vi "RPi_BME280_Raw_Measures_to_Calibrated_Measures_Conversion.vi"(0 "Raw Measures":T1, 5 "Calibration Coefficients":T2) -> (4 "Calibrated Measures":T3)   [LabVIEW 2020]
doc: "Converts Raw Measures to Calibrated Pressure, Temperature and Humidity Measures.\n\nMIT License\nCopyright (c) 2021 Asper"
uses:
  Type_Def/BME280_Calibration_Coefficients.ctl
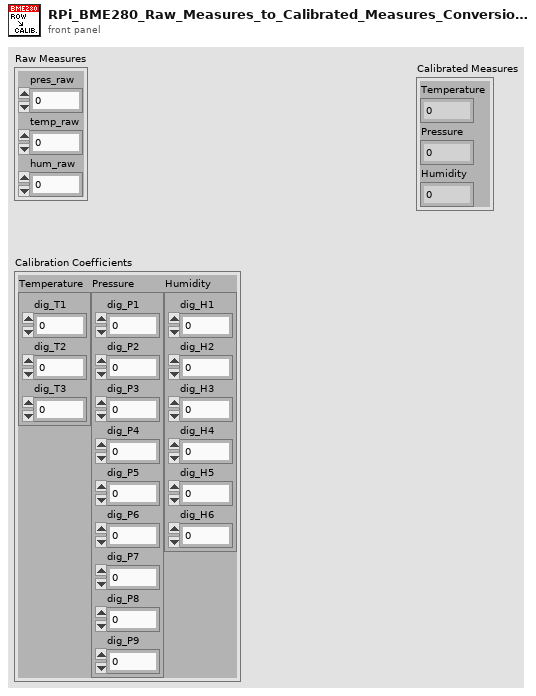
[diagram p1: front panel]
types:
  T1 = cluster{"pres_raw":u32, "temp_raw":u32, "hum_raw":u32}
  T2 = typedef "BME280_Calibration_Coefficients.ctl" = cluster{"Temperature":cluster{"dig_T1":u16, "dig_T2":i16, "dig_T3":i16}, "Pressure":cluster{"dig_P1":u16, "dig_P2":i16, "dig_P3":i16, "dig_P4":i16, "dig_P5":i16, "dig_P6":i16, "dig_P7":i16, "dig_P8":i16, "dig_P9":i16}, "Humidity":cluster{"dig_H1":u8, "dig_H2":i16, "dig_H3":u8, "dig_H4":i16, "dig_H5":i16, "dig_H6":i8}}
  T3 = cluster{"Temperature":dbl, "Pressure":dbl, "Humidity":dbl}
  T4 = cluster{"dig_T1":u16, "dig_T2":i16, "dig_T3":i16}
  T5 = cluster{"dig_H1":u8, "dig_H2":i16, "dig_H3":u8, "dig_H4":i16, "dig_H5":i16, "dig_H6":i8}
  T6 = cluster{"dig_P1":u16, "dig_P2":i16, "dig_P3":i16, "dig_P4":i16, "dig_P5":i16, "dig_P6":i16, "dig_P7":i16, "dig_P8":i16, "dig_P9":i16}
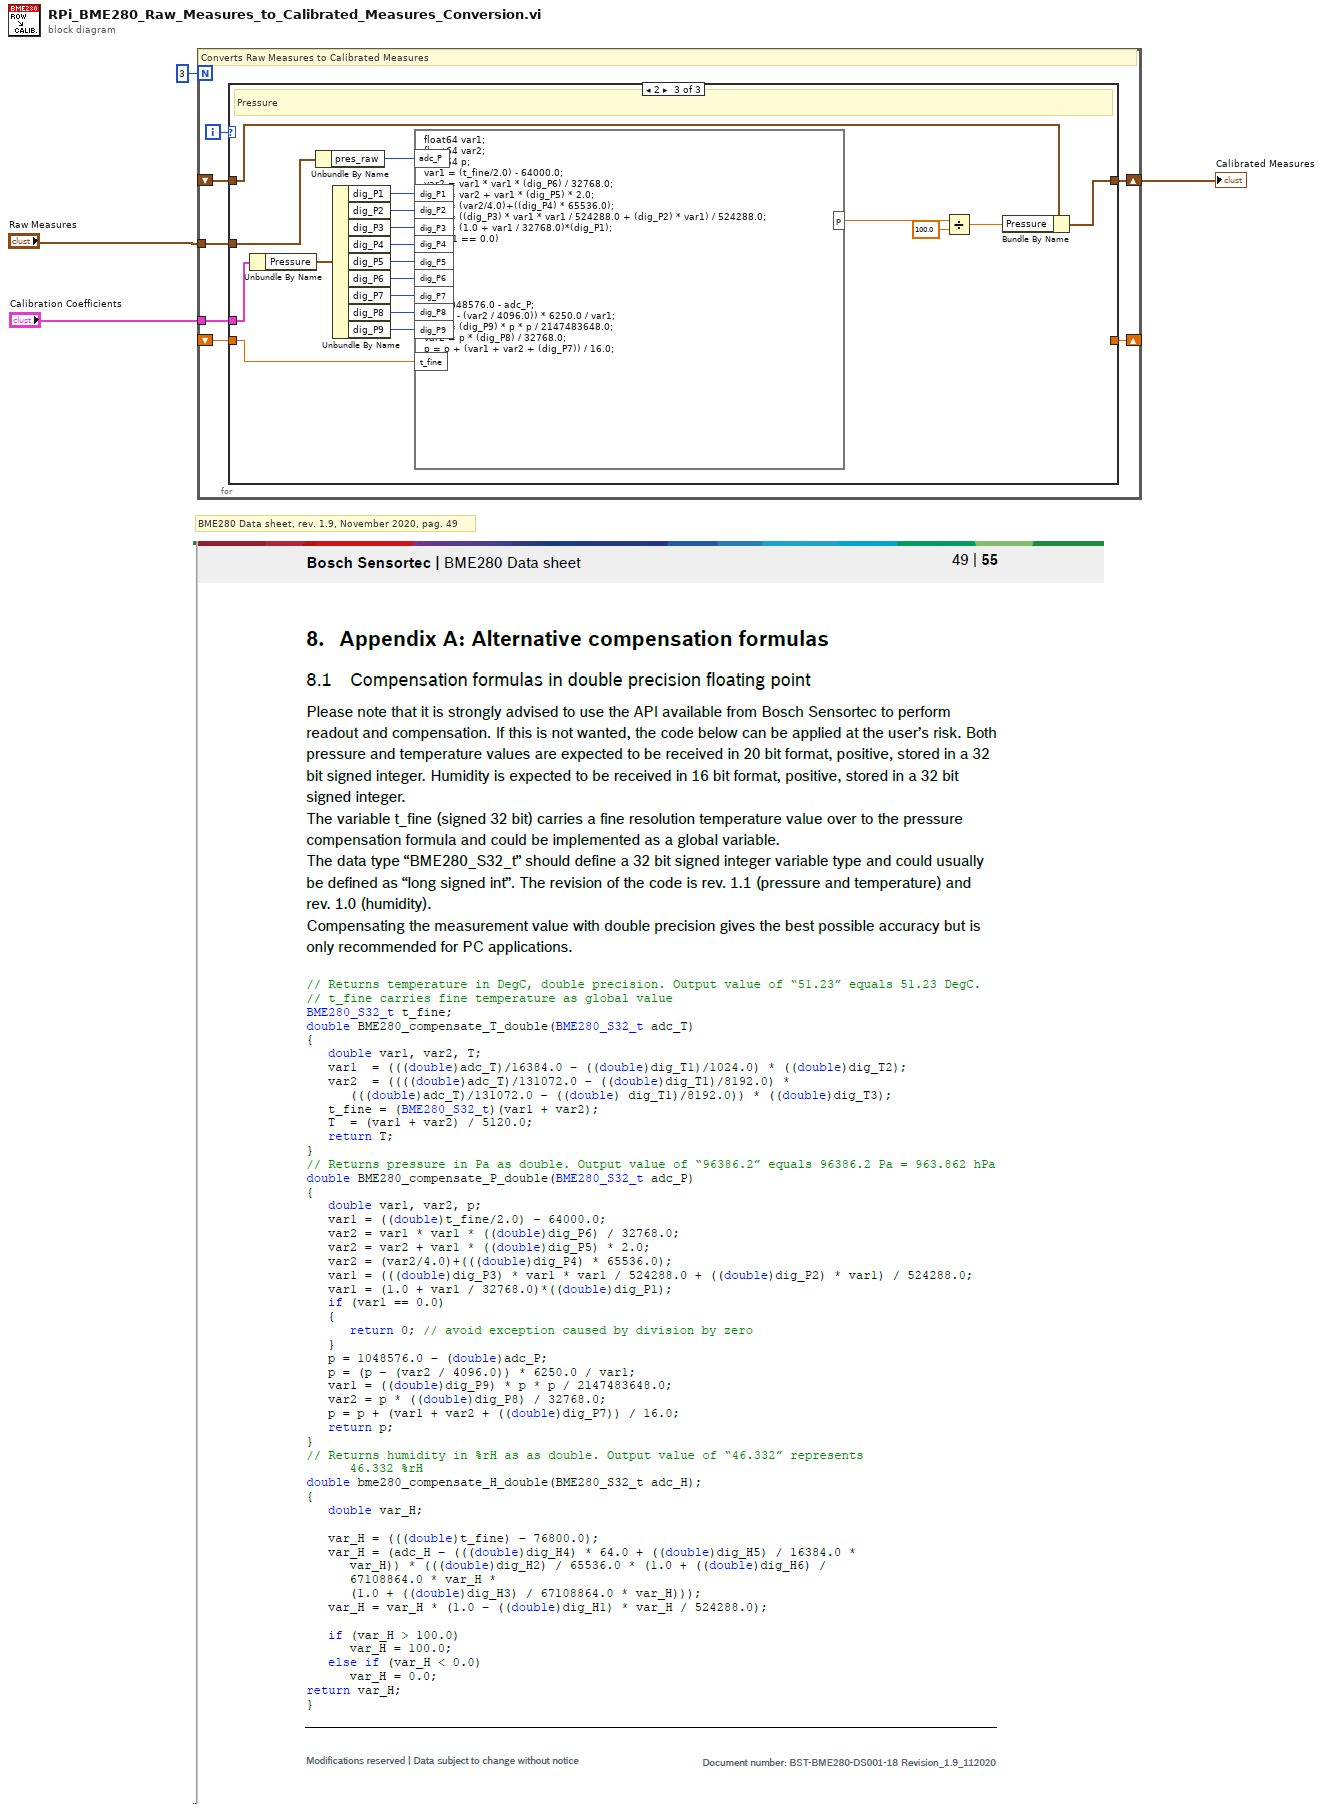
[diagram p0: block diagram]
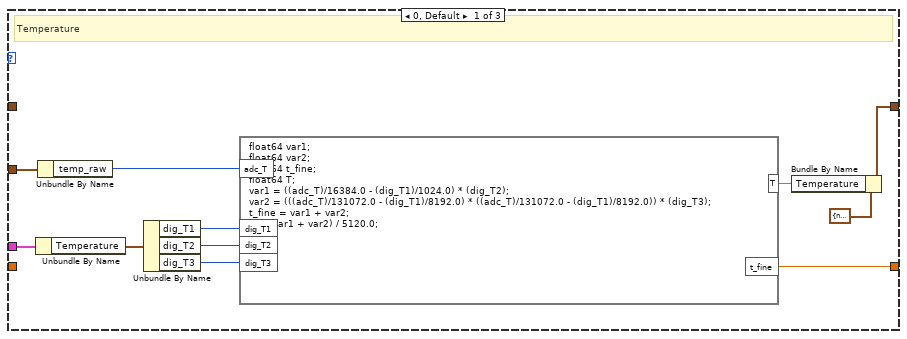
[diagram p2: hidden frame]
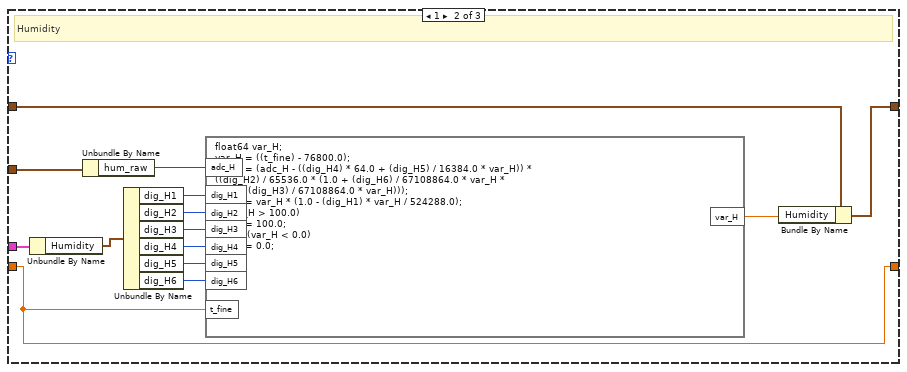
[diagram p3: hidden frame]
diagram:
  # "BME280 Data sheet, rev. 1.9, November 2020, pag. 49"
  n1 = for {
    N: 3 -> [_]
    tunnel: "Raw Measures" -> [w11]
    tunnel: "Calibration Coefficients" -> [w10]
    shift-right: [w8] -> _
    shift-left: _ -> [w7]
    shift-right: [w6] -> w4
    shift-left: _ -> [w5]
    i -> [w9]
    # "Converts Raw Measures to Calibrated Measures"
    n2 = case shown="2" w9 {
      tunnel: w11 -> [w18 w29 w43]
      tunnel: w10 -> [w17 w28 w38]
      tunnel: [w15 w26 _] -> w8
      tunnel: w7 -> [_ w26 w42]
      tunnel: [w12 w23 w39] -> w6
      tunnel: w5 -> [_ w25 w41]
      frame 0, Default {
        # "Temperature"
        n3 = Unbundle By Name(w17) -> ("Temperature"=w16:T4)
        n4 = Unbundle By Name(w18) -> ("temp_raw"=w22:u32)
        n5 = Unbundle By Name(w16) -> ("dig_T1"=w21:u16, "dig_T2"=w20:i16, "dig_T3"=w19:i16)
        n6 = formula code="float64 var1;\nfloat64 var2;\nfloat64 t_fine;\nfloat64 T;\nvar1 = ((adc_T)/16384.0 - (dig_T1)/1024.0) * (dig_T2);\nvar2 = (((adc_T)/131072.0 - (dig_T1)/8192.0) * ((adc_T)/131072.0 - (dig_T1)/8192.0)) * (dig_T3);\nt_fine = var1 + var2;\nT = (var1 + var2) / 5120.0;"("adc_T"=w22, "dig_T1"=w21, "dig_T2"=w20, "dig_T3"=w19) -> ("T"=w13:dbl, "t_fine"=w15:dbl)
        n7 = Bundle By Name(cluster=T3 {"Temperature"=nan, "Pressure"=nan, "Humidity"=nan}, "Temperature"=w13) -> (w12:T3)
      }
      frame 1 {
        # "Humidity"
        n8 = Unbundle By Name(w28) -> ("Humidity"=w27:T5)
        n9 = Unbundle By Name(w29) -> ("hum_raw"=w30:u32)
        n10 = Unbundle By Name(w27) -> ("dig_H1"=w31:u8, "dig_H2"=w32:i16, "dig_H3"=w33:u8, "dig_H4"=w34:i16, "dig_H5"=w35:i16, "dig_H6"=w36:i8)
        n11 = formula code="float64 var_H;\nvar_H = ((t_fine) - 76800.0);\nvar_H = (adc_H - ((dig_H4) * 64.0 + (dig_H5) / 16384.0 * var_H)) *\n((dig_H2) / 65536.0 * (1.0 + (dig_H6) / 67108864.0 * var_H *\n(1.0 + (dig_H3) / 67108864.0 * var_H)));\nvar_H = var_H * (1.0 - (dig_H1) * var_H / 524288.0);\nif (var_H > 100.0)\nvar_H = 100.0;\nelse if (var_H < 0.0)\nvar_H = 0.0;"("adc_H"=w30, "dig_H1"=w31, "dig_H2"=w32, "dig_H3"=w33, "dig_H4"=w34, "dig_H5"=w35, "dig_H6"=w36, "t_fine"=w26) -> ("var_H"=w24:dbl)
        n12 = Bundle By Name(cluster=w25, "Humidity"=w24) -> (w23:T3)
      }
      frame 2 {
        # "Pressure"
        n13 = Unbundle By Name(w38) -> ("Pressure"=w37:T6)
        n14 = Unbundle By Name(w43) -> ("pres_raw"=w45:u32)
        n15 = Unbundle By Name(w37) -> ("dig_P1"=w46:u16, "dig_P2"=w47:i16, "dig_P3"=w48:i16, "dig_P4"=w49:i16, "dig_P5"=w50:i16, "dig_P6"=w51:i16, "dig_P7"=w52:i16, "dig_P8"=w53:i16, "dig_P9"=w54:i16)
        n16 = formula code="float64 var1;\nfloat64 var2;\nfloat64 p;\nvar1 = (t_fine/2.0) - 64000.0;\nvar2 = var1 * var1 * (dig_P6) / 32768.0;\nvar2 = var2 + var1 * (dig_P5) * 2.0;\nvar2 = (var2/4.0)+((dig_P4) * 65536.0);\nvar1 = ((dig_P3) * var1 * var1 / 524288.0 + (dig_P2) * var1) / 524288.0;\nvar1 = (1.0 + var1 / 32768.0)*(dig_P1);\nif (var1 == 0.0)\n{\np = 0;\n}\nelse\n{\np = 1048576.0 - adc_P;\np = (p - (var2 / 4096.0)) * 6250.0 / var1;\nvar1 = (dig_P9) * p * p / 2147483648.0;\nvar2 = p * (dig_P8) / 32768.0;\np = p + (var1 + var2 + (dig_P7)) / 16.0;\n}"("adc_P"=w45, "dig_P1"=w46, "dig_P2"=w47, "dig_P3"=w48, "dig_P4"=w49, "dig_P5"=w50, "dig_P6"=w51, "dig_P7"=w52, "dig_P8"=w53, "dig_P9"=w54, "t_fine"=w42) -> ("p"=w55:dbl)
        n17 = Divide(x=w55, y=100.0) -> (x/y=w40:dbl)
        n18 = Bundle By Name(cluster=w41, "Pressure"=w40) -> (w39:T3)
      }
    }
  }
  "Calibrated Measures" <- w4
